vi "FT_Set_Bit_Mode.vi"(8 "error in (no error)":errorcluster, 9 "Bit Mode":u8(ring) items=["Reset Bit Mode"=0, "Asynchronous Bit Bang"=1, "MPSSE"=2, "Synchronous Bit Bang"=4, "MCU Host Bus Emulation"=8, "Fast Opto-Isolated Serial"=16, "CBUS Bit Bang"=32, "Single Channel 245 Synchronous FIFO"=64], 10 "Bit Mode Mask":u8 format="%x", 11 "Handle In":u64) -> (0 "error out":errorcluster, 1 "FT_Status":u32(ring) items=["FT_OK", "FT_INVALID_HANDLE", "FT_DEVICE_NOT_FOUND", "FT_DEVICE_NOT_OPENED", "FT_IO_ERROR", "FT_INSUFFICIENT_RESOURCES", "FT_INVALID_PARAMETER", "FT_INVALID_BAUD_RATE", "FT_DEVICE_NOT_OPENED_FOR_ERASE", "FT_DEVICE_NOT_OPENED_FOR_WRITE", "FT_FAILED_TO_WRITE_DEVICE", "FT_EEPROM_READ_FAILED", "FT_EEPROM_WRITE_FAILED", "FT_EEPROM_ERASE_FAILED", "FT_EEPROM_NOT_PRESENT", "FT_EEPROM_NOT_PROGRAMMED", "FT_INVALID_ARGS", "FT_NOT_SUPPORTED", "FT_OTHER_ERROR"], 3 "Handle Out":u64)   [LabVIEW 2018]
uses:
  FTD2XX.dll
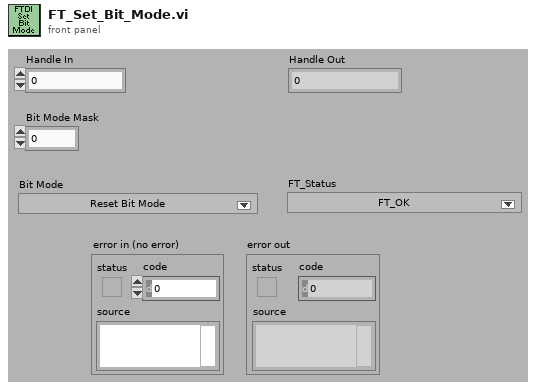
[diagram p1: front panel]
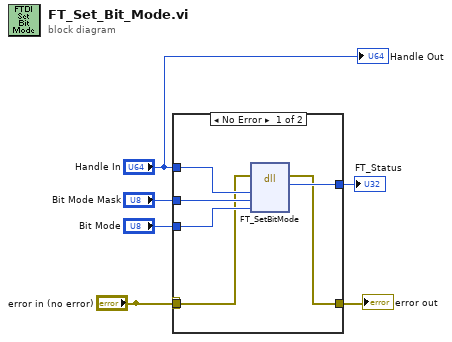
[diagram p0: block diagram]
diagram:
  n1 = case shown="No Error" "error in (no error)" {
    selector: "error in (no error)" -> [_ w13]
    tunnel: "Bit Mode" -> [w12 _]
    tunnel: "Bit Mode Mask" -> [w11 _]
    tunnel: "Handle In" -> [w10 _]
    tunnel: [w9 _] -> w4
    tunnel: [w7 w13] -> w3
    tunnel: "error in (no error)" -> [w8 _]
    frame No Error {
      n2 = dll-call lib="FTD2XX.dll" fn="FT_SetBitMode"(error in=w8, "Handle"=w10, "Mask"=w11, "Enable"=w12) -> (error out=w7:errorcluster, "FT_Status"=w9:u32)  [unwired: 5 in, 1 out]
    }
    frame Error {
    }
  }
  "FT_Status" <- w4
  "error out" <- w3
  "Handle Out" <- "Handle In"
